vi "Phase HS Reset.vi"(8 "Hip Sum":dbl, 9 "Number of Samples":dbl, 11 "Feedback In":T1) -> (0 "Feedback Out":T1)   [LabVIEW 2018]
uses:
  Phase Calculator Feedback Cluster.ctl
  <vilib>/ptbypt/NI_PtbyPt.lvlib
types:
  T1 = typedef "Phase Calculator Feedback Cluster.ctl" = cluster{"k":dbl, "ix0":dbl, "X_max":dbl, "X_min":dbl, "Y_max":dbl, "Y_min":dbl, "Y":dbl, "Hip Sum":dbl, "Num Samples":dbl, "First Heel Strike Done?":bool, "Second Heel Strike Done?":bool, "phi_1":dbl, "phi_end":dbl, "X":dbl}
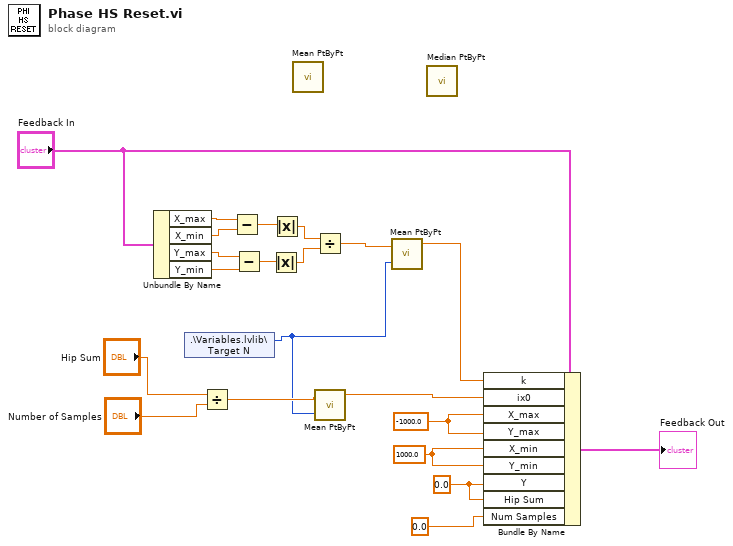
[diagram p0: block diagram]
diagram:
  w19 = 1000.0 ("X_max")
  w20 = -1000.0 ("X_max")
  w21 = 0.0 ("Y")
  n1 = Unbundle By Name("Feedback In") -> ("X_max"=w14:dbl, "X_min"=w13:dbl, "Y_max"=w10:dbl, "Y_min"=w9:dbl)
  n2 = shared-variable ".\\Variables.lvlib\\Target N"() -> (w1:u32)  [unwired: 1 in, 1 out]
  n3 = Divide(x="Hip Sum", y="Number of Samples") -> (x/y=w4:dbl)
  n4 = Subtract(x=w14, y=w13) -> (x-y=w12:dbl)
  n5 = Subtract(x=w10, y=w9) -> (x-y=w11:dbl)
  n6 = Absolute Value(x=w11) -> (abs(x)=w7:dbl)
  n7 = Absolute Value(x=w12) -> (abs(x)=w8:dbl)
  n8 = call <vilib>:"Mean PtByPt.vi"() -> ()  [unwired: 4 in, 2 out]
  n9 = Divide(x=w8, y=w7) -> (x/y=w3:dbl)
  n10 = call <vilib>:"Mean PtByPt.vi"("x"=w4, "sample length"=w1) -> ("mean"=w5:dbl)  [unwired: 2 in, 1 out]
  n11 = call <vilib>:"Mean PtByPt.vi"("x"=w3, "sample length"=w1) -> ("mean"=w2:dbl)  [unwired: 2 in, 1 out]
  n12 = call <vilib>:"Median PtByPt.vi"() -> ()  [unwired: 4 in, 2 out]
  n13 = Bundle By Name(cluster="Feedback In", "k"=w2, "ix0"=w5, "X_max"=w20, "Y_max"=w20, "X_min"=w19, "Y_min"=w19, "Y"=w21, "Hip Sum"=w21, "Num Samples"=0.0) -> (→"Feedback Out":T1)
